vi "get_format_node_term.vi"(0 "Terms[] In":refnum<vi>[](array[refnum]), 5 "Number of Parameters":i32=1, 11 "error in (no error)":errorcluster) -> (4 "Terms[]  Out":refnum<vi>[](array[refnum]), 6 "Format Terms Out":refnum<vi>[](array[refnum]), 15 "error out":errorcluster)   [LabVIEW 2018]
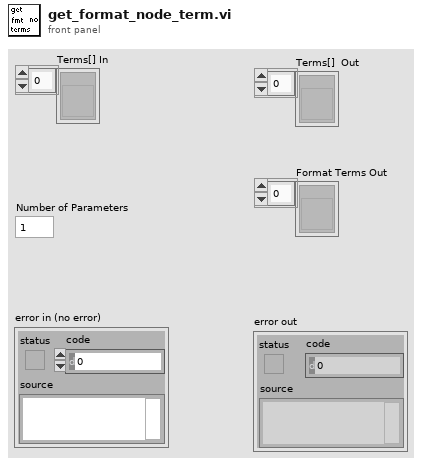
[diagram p1: front panel]
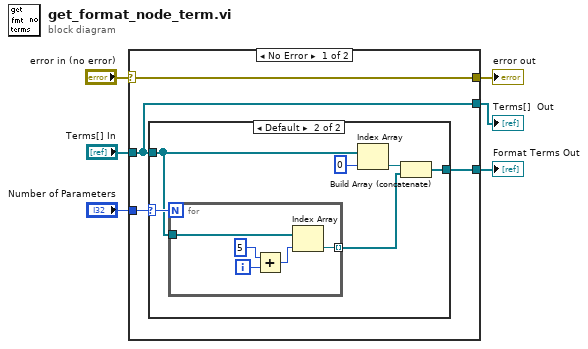
[diagram p0: block diagram]
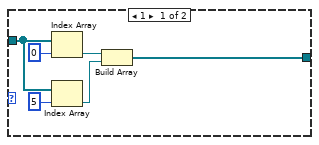
[diagram p2: hidden frame]
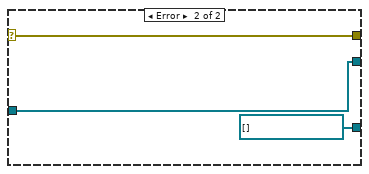
[diagram p3: hidden frame]
diagram:
  n1 = case shown="No Error" "error in (no error)" {
    selector: "error in (no error)" -> [w9 w30]
    tunnel: "Terms[] In" -> [w10 w29]
    tunnel: [w9 w30] -> w4
    tunnel: [w10 w29] -> w3
    tunnel: "Number of Parameters" -> [w8 _]
    tunnel: [w7 refnum<vi>[] []] -> w1
    frame No Error {
      n2 = case shown="Default" w8 {
        selector: w8 -> [_ w22]
        tunnel: w10 -> [w14 w21]
        tunnel: [w11 w17] -> w7
        frame 1 {
          n3 = Index Array(array=w14, index=0) -> (element=w13:refnum<vi>)
          n4 = Index Array(array=w14, index=5) -> (element=w12:refnum<vi>)
          n5 = Build Array(w13, w12) -> (w11:refnum<vi>[])
        }
        frame Default {
          n6 = for {
            N: w22 -> [_]
            tunnel: w21 -> [w24]
            tunnel: [w23] -> w18 mode=indexing
            i -> [w27]
            n7 = Add(x=5, y=w27) -> (x+y=w25:i32)
            n8 = Index Array(array=w24, index=w25) -> (element=w23:refnum<vi>)
          }
          n9 = Index Array(array=w21, index=0) -> (element=w19:refnum<vi>)
          n10 = Build Array (concatenate)(w19, w18) -> (w17:refnum<vi>[])
        }
      }
    }
    frame Error {
    }
  }
  "error out" <- w4
  "Terms[]  Out" <- w3
  "Format Terms Out" <- w1
